vi "RefLevel.vi"(5 "REF 종료점":u16=620, 7 "REF 시작점":u16=320, 8 "거리 배열":dbl[](array[numeric]), 9 "Log(S) 배열":dbl[](array[numeric]), 10 "Log(AS) 배열":dbl[](array[numeric]), 11 "데이터 총량":u32) -> (0 "REF 계산값":dbl, 1 "Log(AS-S)":dbl[](array[numeric]), 2 "REF 스톡스":dbl[](array[numeric]), 3 "REF 안티스톡스":dbl[](array[numeric]), 4 "Log(S) REF":dbl, 6 "Log(AS) REF":dbl)   [LabVIEW 2020]
panel:
  out "XY Graph":cluster{"Y":dbl[], "Y":dbl[]}[](graph) caption="XY 그래프"
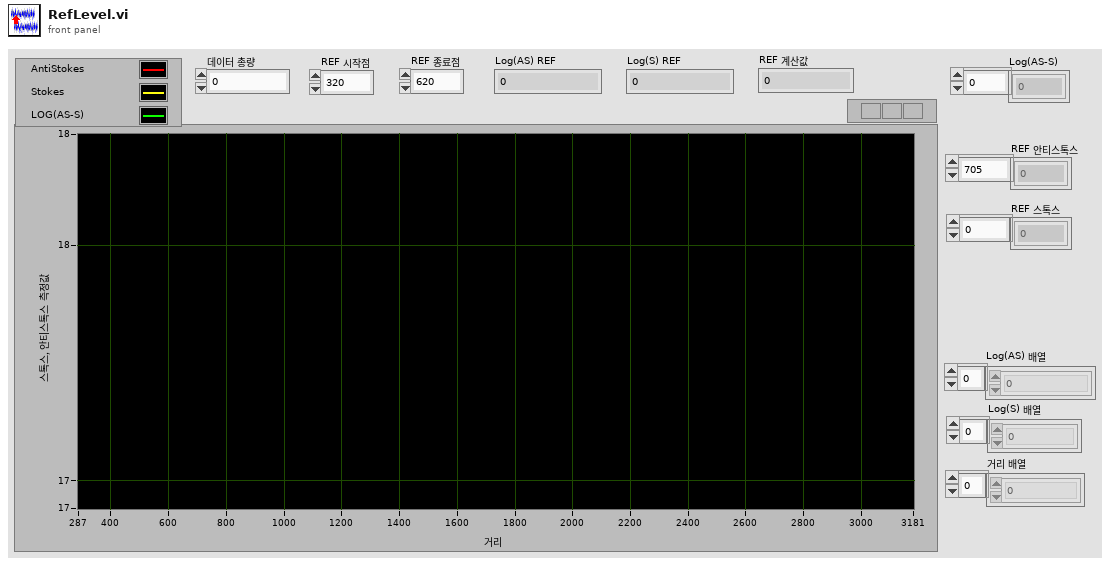
[diagram p1: front panel]
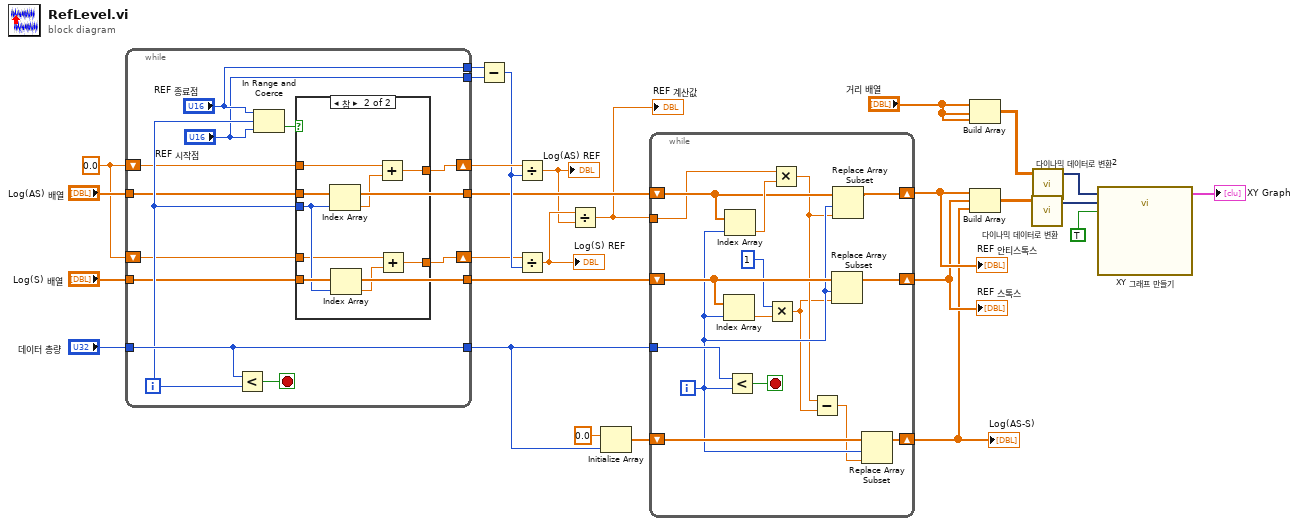
[diagram p0: block diagram]
diagram:
  w20 = 0.0
  n1 = while {
    tunnel: [w39] -> w3
    tunnel: "데이터 총량" -> [w39]
    shift-right: [w34] -> w17
    shift-left: w20 -> [w35]
    shift-right: [w32] -> w15
    shift-left: w20 -> [w33]
    tunnel: "Log(AS) 배열" -> [w31]
    tunnel: [w31] -> w14
    tunnel: "Log(S) 배열" -> [w30]
    tunnel: [w30] -> w13
    tunnel: ["REF 종료점"] -> w19
    tunnel: ["REF 시작점"] -> w18
    i -> [w36]
    stop <- w38 stop-if-true
    n2 = Less?(x=w39, y=w36) -> (x < y?=w38:bool)
    n3 = In Range and Coerce(upper limit="REF 종료점", x=w36, lower limit="REF 시작점") -> (In Range?=w37:bool)  [unwired: 1 out]
    n4 = case shown="참" w37 {
      tunnel: w31 -> [_ w50]
      tunnel: w30 -> [_ w49]
      tunnel: w36 -> [_ w48]
      tunnel: w35 -> [w41 w47]
      tunnel: [w41 w45] -> w34
      tunnel: w33 -> [w40 w44]
      tunnel: [w40 w43] -> w32
      frame False {
      }
      frame True {
        n5 = Index Array(array=w50, index=w48) -> (element=w46:dbl)
        n6 = Index Array(array=w49, index=w48) -> (element=w42:dbl)
        n7 = Add(x=w47, y=w46) -> (x+y=w45:dbl)
        n8 = Add(x=w44, y=w42) -> (x+y=w43:dbl)
      }
    }
  }
  n9 = Subtract(x=w19, y=w18) -> (x-y=w16:u16)
  n10 = Divide(x=w17, y=w16) -> (x/y=w6:dbl)
  "Log(AS) REF" <- w6
  n11 = Divide(x=w15, y=w16) -> (x/y=w7:dbl)
  "Log(S) REF" <- w7
  n12 = Divide(x=w7, y=w6) -> (x/y=w12:dbl)
  "REF 계산값" <- w12
  n13 = Initialize Array(0.0 ("원소"), w3) -> (w5:dbl[])
  n14 = while {
    shift-right: [w59] -> w10
    shift-left: w14 -> [w58]
    shift-right: [w62] -> w9
    shift-left: w13 -> [w63]
    tunnel: w3 -> [w66]
    tunnel: w12 -> [w57]
    shift-right: [w55] -> w1
    shift-left: w5 -> [w56]
    i -> [w54]
    stop <- w65 stop-if-true
    n15 = Index Array(array=w63, index=w54) -> (element=w64:dbl)
    n16 = Index Array(array=w58, index=w54) -> (element=w61:dbl)
    n17 = Less?(x=w66, y=w54) -> (x < y?=w65:bool)
    n18 = Multiply(x=1, y=w64) -> (x*y=w52:dbl)
    n19 = Multiply(x=w57, y=w61) -> (x*y=w53:dbl)
    n20 = Subtract(x=w53, y=w52) -> (x-y=w51:dbl)
    n21 = Replace Array Subset(array=w63, new element=w52, index=w54) -> (w62:dbl[])
    n22 = Replace Array Subset(array=w58, new element=w53, index=w54) -> (w59:dbl[])
    n23 = Replace Array Subset(array=w56, new element=w51, index=w54) -> (w55:dbl[])
  }
  "REF 스톡스" <- w9
  "REF 안티스톡스" <- w10
  "Log(AS-S)" <- w1
  n24 = Build Array("거리 배열", "거리 배열", "거리 배열") -> (w11:dbl[][])
  n25 = Build Array(w10, w9, w1) -> (w8:dbl[][])
  n26 = call "다이나믹 데이터로 변환"("2D Array"=w8) -> ("Dynamic Data Type"=w25:dynamicdata)  [unwired: 3 in]
  n27 = call "다이나믹 데이터로 변환2"("2D Array"=w11) -> ("Dynamic Data Type"=w26:dynamicdata)  [unwired: 3 in]
  n28 = call "XY 그래프 만들기"("Reset"=TRUE, "Y Input"=w25, "X Input"=w26) -> ("XY Graph"=→"XY Graph":cluster{"X":dbl[], "Y":dbl[]}[])  [unwired: 7 in, 1 out]
